vi "TDMS binario.vi"(8 "error in (no error)":errorcluster, 10 "Leds 2":bool[](array[boolean]), 11 "TDMS contador in":refnum<class "TDMS contador.lvclass">) -> (0 "error out":errorcluster, 3 "Login bin out":refnum<class "Login bin.lvclass">)   [LabVIEW 2020, in "TDMS contador.lvlib" / "TDMS contador.lvclass"]
uses:
  TDMS contador.lvclass
  C:/Users/Ceci Saldivar/Desktop/ceci/7mo semestre/Henry/Actor-Tarea-10-12-2020/Login bin/Login bin/Login bin.lvclass
  Login bin/Login bin/Login bin.lvclass
  Login bin/Login bin/Login bin.lvclass/Login bin.ctl
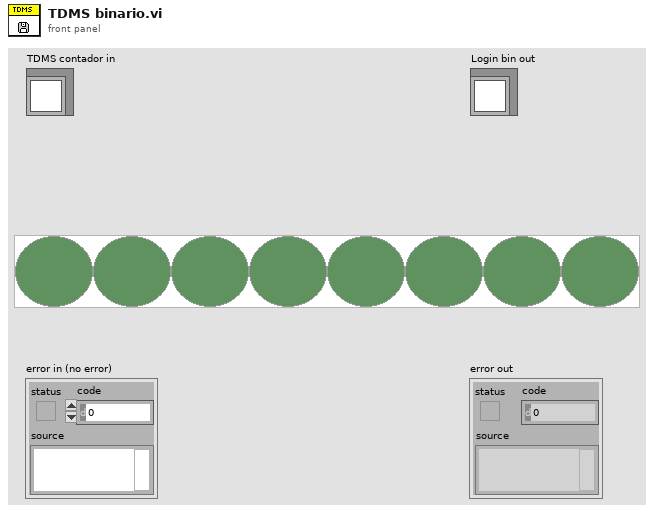
[diagram p1: front panel]
types:
  T1 = enum16{"open", "open or create", "create or replace", "create", "open (read-only)"}
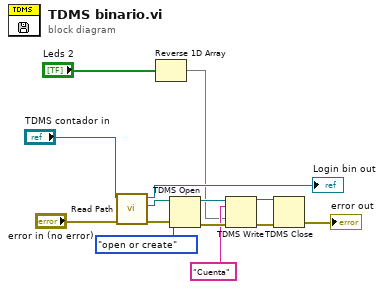
[diagram p0: block diagram]
diagram:
  n1 = call "Read Path.vi"("error in (no error)"="error in (no error)", "Login bin in"="TDMS contador in") -> ("error out"=w12:errorcluster, "Path"=w11:path, "Login bin out"=→"Login bin out":refnum<class "TDMS contador.lvclass">)  [unwired: 7 in]
  n2 = Reverse 1D Array(array="Leds 2") -> (reversed array=w1:bool[])
  n3 = TDMS Open(8:w12, 10:T1."open or create" ("operation (0:open)"), 11:w11) -> (0:w8:errorcluster, 3:w9:refnum<k34>)  [unwired: 4 in]
  n4 = TDMS Write(0:w9, 5:"Cuenta" ("group name in (Untitled)"), 9:w1, 11:w8) -> (4:w5:refnum<k34>, 15:w6:errorcluster)  [unwired: 2 in, 2 out]
  n5 = TDMS Close(8:w6, 11:w5) -> (0:→"error out":errorcluster)  [unwired: 1 out]
